vi "Save As CSV.vi"(8 "error in (no error)":errorcluster caption="错误输入（无错误）", 10 "dup path":path, 11 "从板个数":i32) -> (0 "error out":errorcluster caption="错误输出")   [LabVIEW 2013]
uses:
  <vilib>/Utility/file.llb/Write To Spreadsheet File (string).vi
panel:
  out "充电":bool
  out "预充":bool
  out "总负":bool
  out "总正":bool
  out "风机":bool
  out "加热":bool
  out "DO1":bool
  out "DO2":bool
  out "DI4":bool
  out "DI3":bool
  out "DI2":bool
  out "DI1":bool
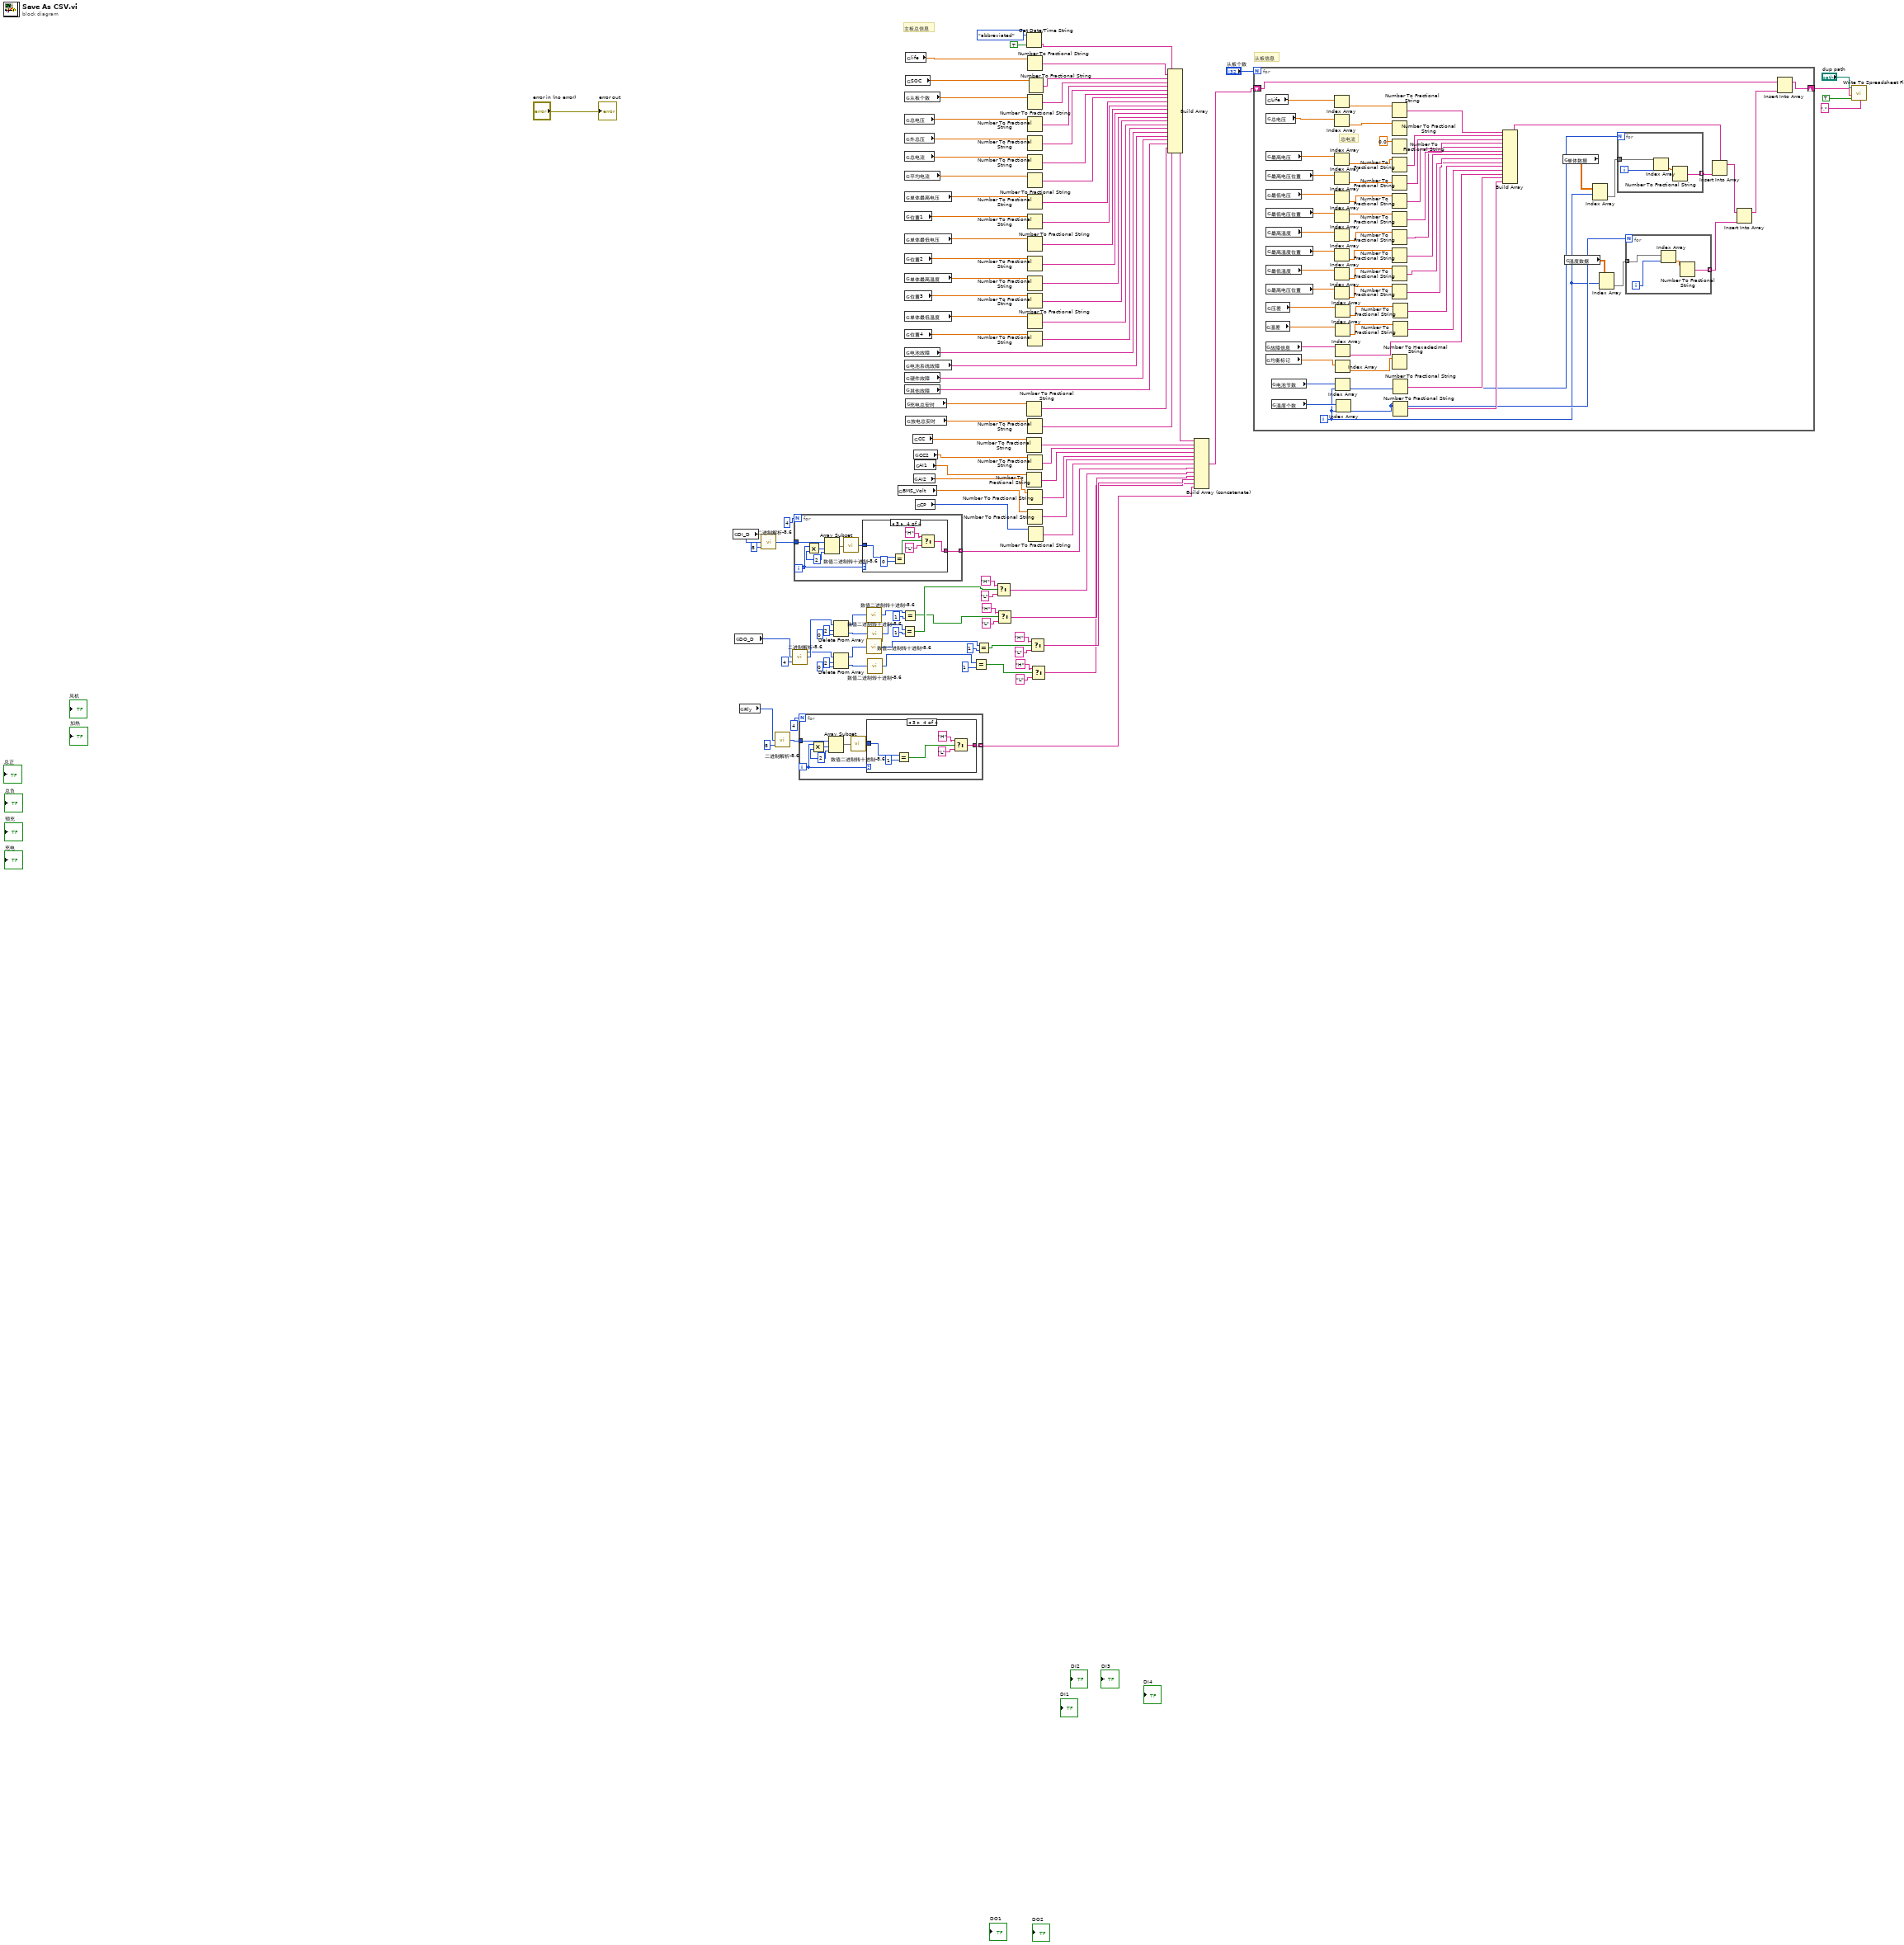
[diagram p0: block diagram]
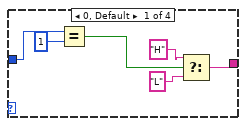
[diagram p2: hidden frame]
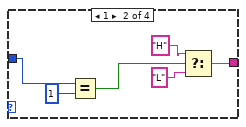
[diagram p3: hidden frame]
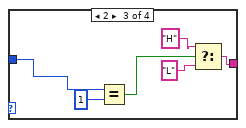
[diagram p4: hidden frame]
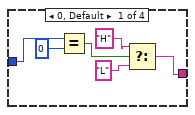
[diagram p5: hidden frame]
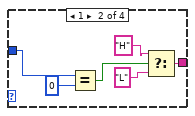
[diagram p6: hidden frame]
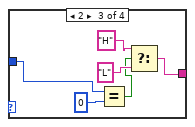
[diagram p7: hidden frame]
diagram:
  # "从板信息"
  # "主板总信息"
  n1 = global read "电池信息全局变量.vi" "DI_D"() -> (w58:u8)
  n2 = global read "电池信息全局变量.vi" "DO_D"() -> (w37:u8)
  n3 = global read "电池信息全局变量.vi" "Rly"() -> (w33:u8)
  n4 = call "二进制解析-8.6.vi"("索引"=8, "数值"=w58) -> ("低位子数组"=w57:i32[])  [unwired: 3 out]
  n5 = call "二进制解析-8.6.vi"("索引"=8, "数值"=w33) -> ("低位子数组"=w36:i32[])  [unwired: 3 out]
  n6 = call "二进制解析-8.6.vi"("索引"=4, "数值"=w37) -> ("低位子数组"=w52:i32[], "高位子数组"=w43:i32[])  [unwired: 2 out]
  n7 = for {
    N: 4 -> [_]
    tunnel: w57 -> [w114]
    tunnel: [w108] -> w18 mode=indexing
    i -> [w110]
    w111 = 2 ("y")
    n8 = Multiply(x=w110, y=w111) -> (x*y=w112:i32)
    n9 = Array Subset(array=w114, index=w112, length=w111) -> (w113:i32[])
    n10 = call "数值二进制转十进制-8.6.vi"("子数组"=w113) -> ("十进制数值"=w109:i32)  [unwired: 4 out]
    n11 = case shown="3" w110 {
      tunnel: w109 -> [w120 w125 w131 w137]
      tunnel: [w115 w121 w128 w133] -> w108
      frame 0, Default {
        n12 = Equal?(x=w120, y=0) -> (x = y?=w118:bool)
        n13 = Select(t="H", s=w118, f="L") -> (s? t:f=w115:string)
      }
      frame 1 {
        n14 = Equal?(x=w125, y=0) -> (x = y?=w122:bool)
        n15 = Select(t="H", s=w122, f="L") -> (s? t:f=w121:string)
      }
      frame 2 {
        n16 = Equal?(x=w131, y=0) -> (x = y?=w127:bool)
        n17 = Select(t="H", s=w127, f="L") -> (s? t:f=w128:string)
      }
      frame 3 {
        n18 = Equal?(x=w137, y=0) -> (x = y?=w134:bool)
        n19 = Select(t="H", s=w134, f="L") -> (s? t:f=w133:string)
      }
    }
  }
  n20 = for {
    N: 4 -> [_]
    tunnel: w36 -> [w145]
    tunnel: [w139] -> w1 mode=indexing
    i -> [w141]
    w142 = 2 ("y")
    n21 = Multiply(x=w141, y=w142) -> (x*y=w143:i32)
    n22 = Array Subset(array=w145, index=w143, length=w142) -> (w144:i32[])
    n23 = call "数值二进制转十进制-8.6.vi"("子数组"=w144) -> ("十进制数值"=w140:i32)  [unwired: 4 out]
    n24 = case shown="3" w141 {
      tunnel: w140 -> [w150 w156 w162 w168]
      tunnel: [w146 w152 w158 w164] -> w139
      frame 0, Default {
        n25 = Equal?(x=w150, y=1) -> (x = y?=w147:bool)
        n26 = Select(t="H", s=w147, f="L") -> (s? t:f=w146:string)
      }
      frame 1 {
        n27 = Equal?(x=w156, y=1) -> (x = y?=w153:bool)
        n28 = Select(t="H", s=w153, f="L") -> (s? t:f=w152:string)
      }
      frame 2 {
        n29 = Equal?(x=w162, y=1) -> (x = y?=w159:bool)
        n30 = Select(t="H", s=w159, f="L") -> (s? t:f=w158:string)
      }
      frame 3 {
        n31 = Equal?(x=w168, y=1) -> (x = y?=w165:bool)
        n32 = Select(t="H", s=w165, f="L") -> (s? t:f=w164:string)
      }
    }
  }
  n33 = Delete From Array(array=w52, length=2 ("长度"), index=0 ("索引")) -> (deleted portion=w49:i32[], array with subset deleted=w48:i32[])
  n34 = Delete From Array(array=w43, length=2 ("长度"), index=0 ("索引")) -> (deleted portion=w41:i32[], array with subset deleted=w42:i32[])
  n35 = call "数值二进制转十进制-8.6.vi"("子数组"=w48) -> ("十进制数值"=w54:i32)  [unwired: 4 out]
  n36 = call "数值二进制转十进制-8.6.vi"("子数组"=w42) -> ("十进制数值"=w47:i32)  [unwired: 4 out]
  n37 = call "数值二进制转十进制-8.6.vi"("子数组"=w49) -> ("十进制数值"=w56:i32)  [unwired: 4 out]
  n38 = call "数值二进制转十进制-8.6.vi"("子数组"=w41) -> ("十进制数值"=w46:i32)  [unwired: 4 out]
  n39 = global read "电池信息全局变量.vi" "BMS_Volt"() -> (w26:dbl)
  n40 = Equal?(x=w56, y=1) -> (x = y?=w13:bool)
  n41 = Equal?(x=w54, y=1) -> (x = y?=w12:bool)
  n42 = global read "电池信息全局变量.vi" "从板个数"() -> (w80:dbl)
  n43 = global read "EV05全局变量1.vi" "总电压"() -> (w86:dbl)
  n44 = global read "电池信息全局变量.vi" "外总压"() -> (w84:dbl)
  n45 = global read "EV05全局变量1.vi" "总电流"() -> (w85:dbl)
  n46 = global read "电池信息全局变量.vi" "平均电流"() -> (w83:dbl)
  n47 = global read "EV05全局变量1.vi" "单体最高电压"() -> (w77:dbl)
  n48 = global read "EV05全局变量1.vi" "位置1"() -> (w76:dbl)
  n49 = global read "EV05全局变量1.vi" "单体最低电压"() -> (w75:dbl)
  n50 = global read "EV05全局变量1.vi" "位置2"() -> (w74:dbl)
  n51 = global read "EV05全局变量1.vi" "单体最高温度"() -> (w73:dbl)
  n52 = global read "EV05全局变量1.vi" "位置3"() -> (w72:dbl)
  n53 = global read "EV05全局变量1.vi" "单体最低温度"() -> (w71:dbl)
  n54 = global read "EV05全局变量1.vi" "位置4"() -> (w70:dbl)
  n55 = global read "EV05全局变量1.vi" "电池故障"() -> (w69:string)
  n56 = global read "EV05全局变量1.vi" "电池系统故障"() -> (w68:string)
  n57 = global read "EV05全局变量1.vi" "硬件故障"() -> (w67:string)
  n58 = global read "EV05全局变量1.vi" "其他故障"() -> (w66:string)
  n59 = global read "电池信息全局变量.vi" "充电总安时"() -> (w64:dbl)
  n60 = global read "EV05全局变量1.vi" "life"() -> (w79:dbl)
  n61 = global read "EV05全局变量1.vi" "SOC"() -> (w78:dbl)
  n62 = global read "电池信息全局变量.vi" "放电总安时"() -> (w65:dbl)
  n63 = global read "电池信息全局变量.vi" "CC"() -> (w30:dbl)
  n64 = global read "电池信息全局变量.vi" "AI2"() -> (w27:dbl)
  n65 = global read "电池信息全局变量.vi" "CC2"() -> (w29:dbl)
  n66 = global read "电池信息全局变量.vi" "AI1"() -> (w28:dbl)
  n67 = global read "电池信息全局变量.vi" "CP"() -> (w25:u8)
  n68 = Equal?(x=w46, y=1) -> (x = y?=w4:bool)
  n69 = Equal?(x=w47, y=1) -> (x = y?=w5:bool)
  n70 = Select(t="H", s=w13, f="L") -> (s? t:f=w11:string)
  n71 = Select(t="H", s=w12, f="L") -> (s? t:f=w10:string)
  n72 = Get Date/Time String(date format (0)=enum16{"short", "long", "abbreviated"}."abbreviated" ("日期格式(0)"), want seconds? (F)=TRUE ("需要秒？(F)")) -> (time string=w105:string)  [unwired: 1 in, 1 out]
  n73 = Number To Fractional String(number=w64) -> (F-format string=w88:string)  [unwired: 3 in]
  n74 = Number To Fractional String(number=w30) -> (F-format string=w24:string)  [unwired: 3 in]
  n75 = Number To Fractional String(number=w28) -> (F-format string=w22:string)  [unwired: 3 in]
  n76 = Number To Fractional String(number=w79) -> (F-format string=w63:string)  [unwired: 3 in]
  n77 = Number To Fractional String(number=w65) -> (F-format string=w87:string)  [unwired: 3 in]
  n78 = Number To Fractional String(number=w29) -> (F-format string=w23:string)  [unwired: 3 in]
  n79 = Number To Fractional String(number=w27) -> (F-format string=w21:string)  [unwired: 3 in]
  n80 = Number To Fractional String(number=w80) -> (F-format string=w104:string)  [unwired: 3 in]
  n81 = Number To Fractional String(number=w86) -> (F-format string=w103:string)  [unwired: 3 in]
  n82 = Number To Fractional String(number=w84) -> (F-format string=w82:string)  [unwired: 3 in]
  n83 = Number To Fractional String(number=w85) -> (F-format string=w102:string)  [unwired: 3 in]
  n84 = Number To Fractional String(number=w83) -> (F-format string=w81:string)  [unwired: 3 in]
  n85 = Number To Fractional String(number=w77) -> (F-format string=w100:string)  [unwired: 3 in]
  n86 = Number To Fractional String(number=w76) -> (F-format string=w99:string)  [unwired: 3 in]
  n87 = Number To Fractional String(number=w75) -> (F-format string=w98:string)  [unwired: 3 in]
  n88 = Number To Fractional String(number=w74) -> (F-format string=w97:string)  [unwired: 3 in]
  n89 = Number To Fractional String(number=w73) -> (F-format string=w92:string)  [unwired: 3 in]
  n90 = Number To Fractional String(number=w72) -> (F-format string=w91:string)  [unwired: 3 in]
  n91 = Number To Fractional String(number=w71) -> (F-format string=w90:string)  [unwired: 3 in]
  n92 = Number To Fractional String(number=w70) -> (F-format string=w89:string)  [unwired: 3 in]
  n93 = Number To Fractional String(number=w26) -> (F-format string=w20:string)  [unwired: 3 in]
  n94 = Number To Fractional String(number=w25) -> (F-format string=w19:string)  [unwired: 3 in]
  n95 = Number To Fractional String(number=w78) -> (F-format string=w62:string)  [unwired: 3 in]
  n96 = Select(t="H", s=w5, f="L") -> (s? t:f=w3:string)
  n97 = Select(t="H", s=w4, f="L") -> (s? t:f=w2:string)
  n98 = Build Array(w105, w63, w62, w104, w103, w82, w102, w81, w100, w99, w98, w97, w92, w91, w90, w89, w69, w68, w67, w66, w88, w87) -> (w32:string[])
  n99 = Build Array (concatenate)(w32, w24, w23, w22, w21, w20, w19, w18, w11, w10, w3, w2, w1) -> (w31:string[])
  n100 = for {
    N: "从板个数" -> [_]
    shift-right: [w213] -> w96
    shift-left: w31 -> [w212]
    i -> [w170]
    # "总电流"
    n101 = global read "从板全局变量.vi" "温差"() -> (w182:dbl[])
    n102 = global read "从板全局变量.vi" "故障信息"() -> (w179:string[])
    n103 = global read "从板全局变量.vi" "均衡标记"() -> (w177:dbl[])
    n104 = global read "从板全局变量.vi" "Life"() -> (w205:dbl[])
    n105 = global read "从板全局变量.vi" "总电压"() -> (w203:dbl[])
    n106 = global read "从板全局变量.vi" "最高电压"() -> (w199:dbl[])
    n107 = global read "从板全局变量.vi" "最高电压位置"() -> (w200:dbl[])
    n108 = global read "从板全局变量.vi" "最低电压"() -> (w201:dbl[])
    n109 = global read "从板全局变量.vi" "最低电压位置"() -> (w198:dbl[])
    n110 = global read "从板全局变量.vi" "最高温度"() -> (w197:dbl[])
    n111 = global read "从板全局变量.vi" "最高温度位置"() -> (w196:dbl[])
    n112 = global read "从板全局变量.vi" "最低温度"() -> (w194:dbl[])
    n113 = global read "从板全局变量.vi" "最高电压位置"() -> (w195:dbl[])
    n114 = global read "从板全局变量.vi" "压差"() -> (w183:dbl[])
    n115 = global read "从板全局变量.vi" "电池节数"() -> (w208:u8[])
    n116 = global read "从板全局变量.vi" "温度个数"() -> (w209:u8[])
    n117 = Index Array(array=w205) -> (element=w204:dbl)  [unwired: 1 in]
    n118 = Index Array(array=w203) -> (element=w202:dbl)  [unwired: 1 in]
    n119 = Index Array(array=w199) -> (element=w193:dbl)  [unwired: 1 in]
    n120 = Index Array(array=w200) -> (element=w192:dbl)  [unwired: 1 in]
    n121 = Index Array(array=w201) -> (element=w191:dbl)  [unwired: 1 in]
    n122 = Index Array(array=w198) -> (element=w190:dbl)  [unwired: 1 in]
    n123 = Index Array(array=w197) -> (element=w189:dbl)  [unwired: 1 in]
    n124 = Index Array(array=w196) -> (element=w188:dbl)  [unwired: 1 in]
    n125 = Index Array(array=w194) -> (element=w187:dbl)  [unwired: 1 in]
    n126 = Index Array(array=w195) -> (element=w186:dbl)  [unwired: 1 in]
    n127 = Index Array(array=w183) -> (element=w184:dbl)  [unwired: 1 in]
    n128 = Index Array(array=w182) -> (element=w185:dbl)  [unwired: 1 in]
    n129 = Index Array(array=w179) -> (element=w178:string)  [unwired: 1 in]
    n130 = Index Array(array=w177) -> (element=w176:dbl)  [unwired: 1 in]
    n131 = Index Array(array=w208, index=w170) -> (element=w207:u8)
    n132 = Index Array(array=w209, index=w170) -> (element=w206:u8)
    n133 = Number To Fractional String(number=w204) -> (F-format string=w210:string)  [unwired: 3 in]
    n134 = Number To Fractional String(number=w202) -> ()  [unwired: 3 in, 1 out]
    n135 = Number To Fractional String(number=0.0 ("数字")) -> ()  [unwired: 3 in, 1 out]
    n136 = Number To Fractional String(number=w193) -> (F-format string=w227:string)  [unwired: 3 in]
    n137 = Number To Fractional String(number=w192) -> (F-format string=w226:string)  [unwired: 3 in]
    n138 = Number To Fractional String(number=w191) -> (F-format string=w225:string)  [unwired: 3 in]
    n139 = Number To Fractional String(number=w190) -> (F-format string=w224:string)  [unwired: 3 in]
    n140 = Number To Fractional String(number=w189) -> (F-format string=w223:string)  [unwired: 3 in]
    n141 = Number To Fractional String(number=w188) -> (F-format string=w222:string)  [unwired: 3 in]
    n142 = Number To Fractional String(number=w187) -> (F-format string=w221:string)  [unwired: 3 in]
    n143 = Number To Fractional String(number=w186) -> (F-format string=w220:string)  [unwired: 3 in]
    n144 = Number To Hexadecimal String(2:w176) -> ()  [unwired: 1 in, 1 out]
    n145 = Number To Fractional String(number=w184) -> (F-format string=w181:string)  [unwired: 3 in]
    n146 = Number To Fractional String(number=w185) -> (F-format string=w180:string)  [unwired: 3 in]
    n147 = Number To Fractional String(number=w206) -> (F-format string=w218:string)  [unwired: 3 in]
    n148 = Number To Fractional String(number=w207) -> (F-format string=w219:string)  [unwired: 3 in]
    n149 = Build Array(w210, w227, w226, w225, w224, w223, w222, w221, w220, w181, w180, w178, w219, w218) -> (w216:string[])
    n150 = global read "单体信息全局.vi" "单体数据"() -> (w174:dbl[][])
    n151 = global read "单体信息全局.vi" "温度数据"() -> (w172:sgl[][])
    n152 = Index Array(array=w174, index (row)=w170) -> (element=w173:dbl[])  [unwired: 1 in]
    n153 = Index Array(array=w172, index (row)=w170) -> (element=w171:sgl[])  [unwired: 1 in]
    n154 = for {
      N: w207 -> [_]
      tunnel: [w235] -> w217 mode=indexing
      tunnel: w173 -> [w234]
      i -> [w232]
      n155 = Index Array(array=w234, index=w232) -> (element=w233:dbl)
      n156 = Number To Fractional String(number=w233) -> (F-format string=w235:string)  [unwired: 3 in]
    }
    n157 = for {
      N: w206 -> [_]
      tunnel: [w231] -> w215 mode=indexing
      tunnel: w171 -> [w229]
      i -> [w228]
      n158 = Index Array(array=w229, index=w228) -> (element=w230:sgl)
      n159 = Number To Fractional String(number=w230) -> (F-format string=w231:string)  [unwired: 3 in]
    }
    n160 = Insert Into Array(array=w216, new element=w217) -> (w214:string[])  [unwired: 1 in]
    n161 = Insert Into Array(array=w214, new element=w215) -> (w211:string[])  [unwired: 1 in]
    n162 = Insert Into Array(array=w212, new element=w211) -> (w213:string[])  [unwired: 1 in]
  }
  n163 = call-poly <vilib>:"Write To Spreadsheet File.vi"("delimiter (\\t)"="," ("delimiter (\\t)"), "append to file? (new file:F)"=TRUE, "1D data"=w96, "file path (dialog if empty)"="dup path") -> ()  [unwired: 4 in, 1 out]
  "error out" <- "error in (no error)"
